vi "Actor Core.vi"(8 "error in":errorcluster, 11 "Configuration in":refnum<class "Configuration.lvclass">) -> (0 "error out":errorcluster, 3 "Actor out":refnum<class "Actor.lvclass">)   [LabVIEW 2016, in "Configuration.lvlib" / "Configuration.lvclass"]
doc: "(<B>Filename</B>: Actor Framework.lvlib:Actor.lvclass:Actor Core.vi)\n\nReceives messages to the actor, reacts to them, and initiates any error handling that may shut the actor down.\n\nDescendant classes may override this VI to append parallel tasks for the actor to complete while it handles messages. Overrides use the Call Parent Method node."
uses:
  Configuration.lvclass
  C:/Program Files (x86)/National Instruments/LabVIEW 2016/vi.lib/ActorFramework/Actor/Actor.lvclass
  <vilib>/ActorFramework/Actor/Actor.lvclass
  Config Actor Core UI Ref.ctl
  <vilib>/ActorFramework/Actor/Actor.lvclass/Actor.ctl
  <vilib>/ActorFramework/Message Enqueuer/Message Enqueuer.lvclass/Message Enqueuer.ctl
  Configuration Messages/Display New Configuration SubPanel Msg/Display New Configuration SubPanel Msg.lvclass/Display New Configuration SubPanel Msg.ctl
  Configuration.lvclass/Configuration.ctl
  <vilib>/ActorFramework/Message Enqueuer/Init from Existing Queue.vi
  <vilib>/ActorFramework/Message Enqueuer/Enqueue.vi
  <vilib>/ActorFramework/Stop Msg/Stop Msg.lvclass
  C:/Program Files (x86)/National Instruments/LabVIEW 2016/vi.lib/ActorFramework/Message/Message.lvclass
  Configuration Messages/Display New Configuration SubPanel Msg/Display New Configuration SubPanel Msg.lvclass
  Configuration Messages/Display Help for Selected Category Msg/Display Help for Highlighted Category Msg.lvclass
  <vilib>/ActorFramework/Message Priority Queue/Priority Enqueue.vi
  <vilib>/ActorFramework/Message Enqueuer/Message Enqueuer.lvclass
panel:
  in  "Categories":i32(listbox)
  out "Title":string
  in  "Help":bool
  in  "OK":bool
  in  "Cancel":bool
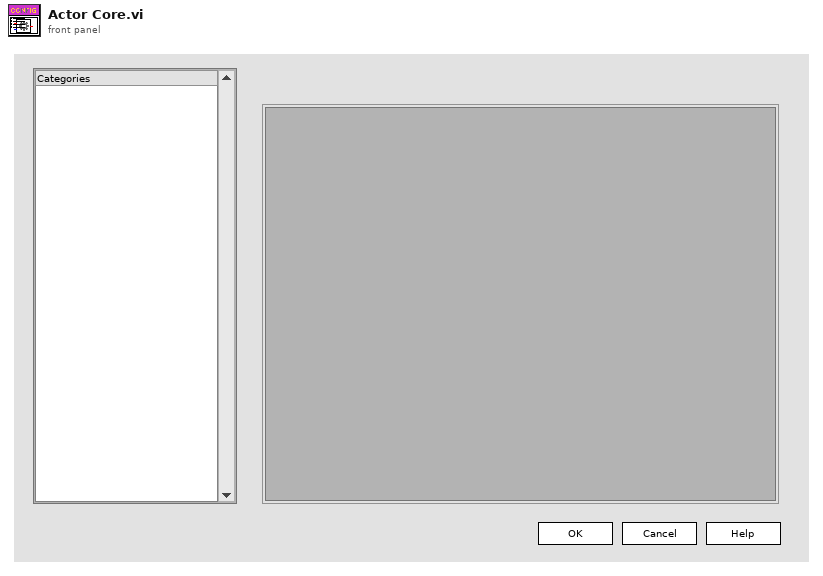
[diagram p1: front panel]
types:
  T1 = typedef "Configuration.lvlib/Configuration.lvclass/Config Actor Core UI Ref.ctl" = cluster{"Title":refnum<vi>, "Sub Panel":refnum<vi>, "OK":refnum<vi>, "Categories":refnum<vi>, "Help":refnum<vi>}
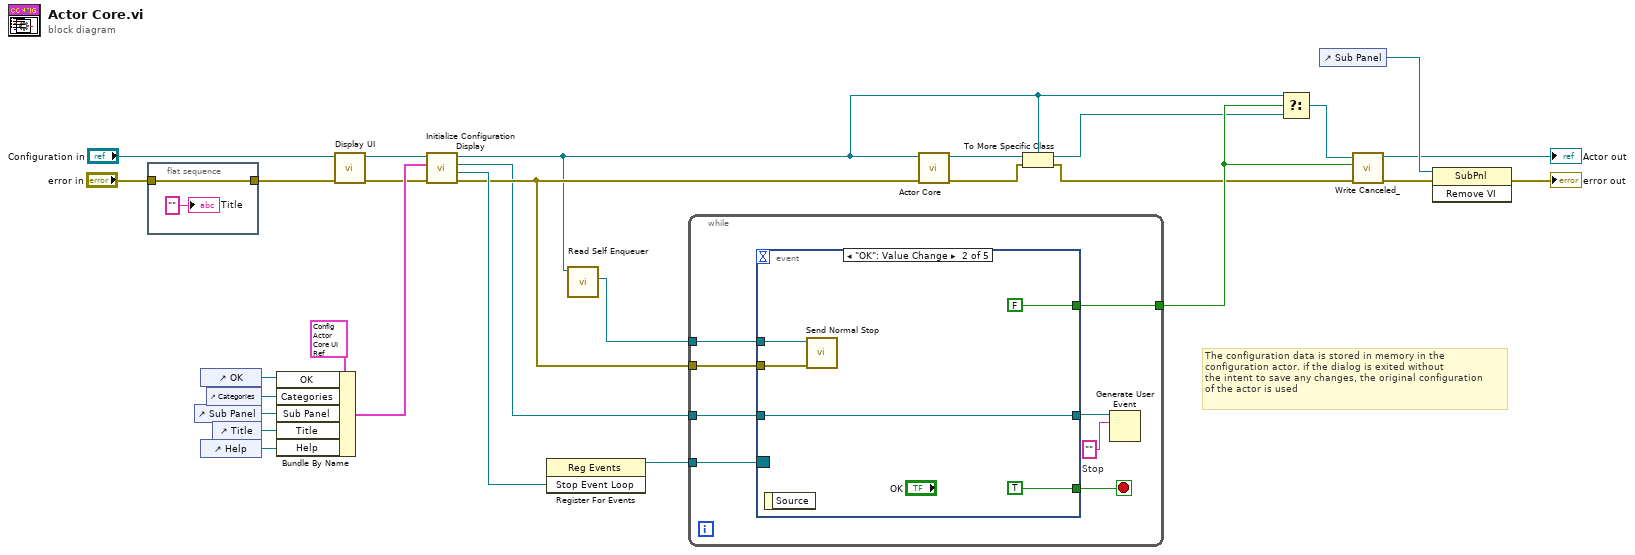
[diagram p0: block diagram]
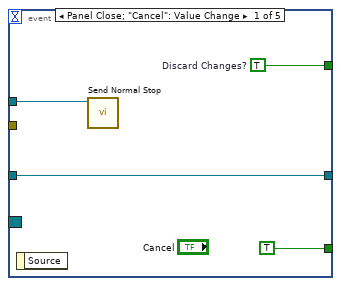
[diagram p2: hidden frame]
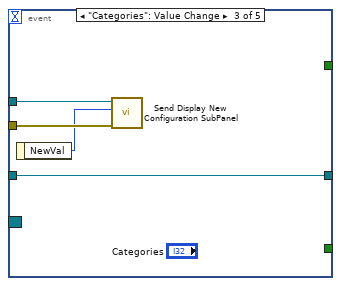
[diagram p3: hidden frame]
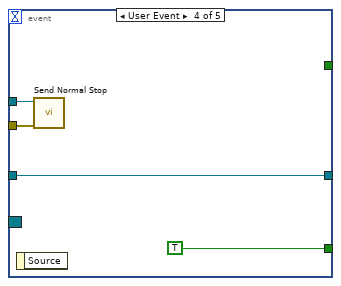
[diagram p4: hidden frame]
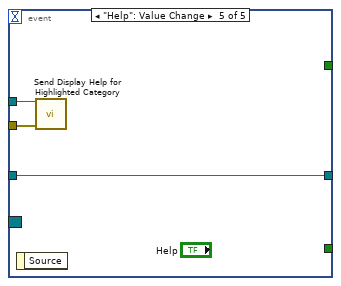
[diagram p5: hidden frame]
diagram:
  # "The configuration data is stored in memory in the\nconfiguration actor. if the dialog is exited without\nthe intent to save any changes, the original configuration\nof the actor is used"
  n1 = flat-sequence {
    tunnel: "error in" -> [w30]
    tunnel: [w30] -> w12
    frame #0 {
      "Title" <- "" ("Title")
    }
  }
  n2 = control-ref of="Sub Panel"() -> (w16:refnum<vi>)
  n3 = control-ref of="OK"() -> (w18:refnum<vi>)
  n4 = control-ref of="Help"() -> (w14:refnum<vi>)
  n5 = control-ref of="Categories"() -> (w17:refnum<vi>)
  n6 = control-ref of="Title"() -> (w15:refnum<vi>)
  n7 = Bundle By Name(cluster=T1 {"Title"=refnum, "Sub Panel"=refnum, "OK"=refnum, "Categories"=refnum, "Help"=refnum} ("Configuration Pane References"), "OK"=w18, "Categories"=w17, "Sub Panel"=w16, "Title"=w15, "Help"=w14) -> (w19:T1)
  n8 = call "Display UI.vi"("error in (no error)"=w12, "Configuration in"="Configuration in") -> ("error out"=w10:errorcluster, "Configuration out"=w11:refnum<class "Configuration.lvclass">)  [unwired: 8 in]
  n9 = call "Initialize Configuration Display.vi"("error in (no error)"=w10, "Configuration Pane References"=w19, "Configuration in"=w11) -> ("error out"=w25:errorcluster, "Stop Event Loop"=w27:refnum<user-event>, "Change Display"=w24:refnum<user-event>, "Configuration out"=w6:refnum<class "Configuration.lvclass">)  [unwired: 5 in]
  n10 = register-events(w27) -> (reference out=w28:refnum<event-registration>)  [unwired: 2 in, 1 out]
  n11 = call <vilib>:"Read Self Enqueuer.vi"("Actor"=w6) -> ("Self Enqueuer"=w26:refnum<class "Message Enqueuer.lvclass">)  [unwired: 10 in]
  n12 = while {
    tunnel: w28 -> [w38]
    tunnel: w26 -> [w36]
    tunnel: w25 -> [w35]
    tunnel: w24 -> [w34]
    tunnel: [w31] -> w9
    stop <- w37 stop-if-true
    w32 = ""  # Stop
    n13 = event shown="[1] \"OK\": Value Change" {
      selector: w38 -> [_ _ _ _ _]
      dyn-events: _ -> [_ _ _ _ _]
      timeout: _ -> [_ _ _ _ _]
      tunnel: [TRUE TRUE _ TRUE _] -> w37
      tunnel: w36 -> [w42 w45 w50 w52 w57]
      tunnel: w35 -> [_ w44 w51 w53 w56]
      tunnel: [w41 w47 w49 w54 w58] -> w33
      tunnel: w34 -> [w41 w47 w49 w54 w58]
      tunnel: [w39 FALSE ("Discard Changes?") _ _ _] -> w31
      event Panel Close; "Cancel": Value Change {
        w39 = TRUE  # Discard Changes?
        n14 = event-data() -> ()  [unwired: 1 in, 1 out]
        n15 = call <vilib>:"Send Normal Stop.vi"("Message Enqueuer"=w42) -> ()  [unwired: 10 in, 1 out]
      }
      event "OK": Value Change {
        n16 = event-data() -> ()  [unwired: 1 in, 1 out]
        n17 = call <vilib>:"Send Normal Stop.vi"("error in (no error)"=w44, "Message Enqueuer"=w45) -> ()  [unwired: 9 in, 1 out]
      }
      event "Categories": Value Change {
        n18 = event-data() -> ("NewVal"=w48:i32)  [unwired: 1 in]
        n19 = call "Send Display New Configuration SubPanel.vi"("error in (no error)"=w51, "ListBox Selection"=w48, "Message Enqueuer"=w50) -> ()  [unwired: 7 in, 2 out]
      }
      event User Event {
        n20 = event-data() -> ()  [unwired: 1 in, 1 out]
        n21 = call <vilib>:"Send Normal Stop.vi"("error in (no error)"=w53, "Message Enqueuer"=w52) -> ()  [unwired: 9 in, 1 out]
      }
      event "Help": Value Change {
        n22 = event-data() -> ()  [unwired: 1 in, 1 out]
        n23 = call "Send Display Help for Highlighted Category.vi"("error in (no error)"=w56, "Message Enqueuer"=w57) -> ()  [unwired: 8 in, 2 out]
      }
    }
    n24 = Generate User Event(user event=w33, event data cluster=w32) -> ()  [unwired: 2 in, 2 out]
  }
  n25 = call-parent "Actor Core.vi"("error in"=w25, "Actor in"=w6) -> ("error out"=w4:errorcluster, "Actor out"=w7:refnum<class "Actor.lvclass">)  [unwired: 8 in]
  n26 = To More Specific Class(target class=w6, reference=w7, error in=w4) -> (specific class reference=w5:refnum<class "Configuration.lvclass">, error out=w3:errorcluster)
  n27 = Select(t=w6, s=w9, f=w5) -> (s? t:f=w2:refnum<class "Configuration.lvclass">)
  n28 = control-ref of="Sub Panel"() -> (w22:refnum<vi>)
  n29 = call "Write Canceled_.vi"("error in (no error)"=w3, "Canceled?"=w9, "Configuration in"=w2) -> ("error out"=w8:errorcluster, "Configuration out"=→"Actor out":refnum<class "Configuration.lvclass">)  [unwired: 7 in]
  n30 = invoke class="SubPnl" method="Remove VI"(reference=w22, error in=w8) -> (error out=→"error out":errorcluster)  [unwired: 1 in, 2 out]
